vi "geterrormessages.vi"(8 "error in (no error)":errorcluster, 11 "hObject":i32=1) -> (0 "error out":errorcluster, 1 "pNumOfErrors":i32, 2 "pErrorMsgs":i32[](array[numeric]), 3 "hObject Out":i32=1)   [LabVIEW 2018]
doc: "This VI returns the errors from the neoVI error queue. Use \"GetErrorInfo\" to return the actual error info.\n\n12/21/2010 1.0.0 jyg\n- initial release"
uses:
  icsneo40.dll
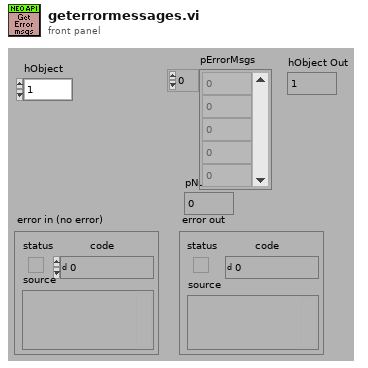
[diagram p1: front panel]
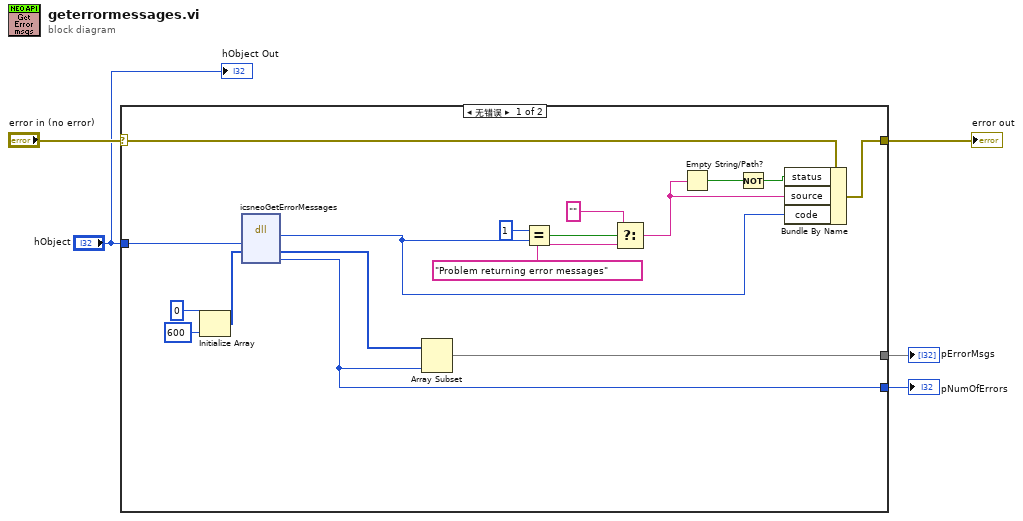
[diagram p0: block diagram]
diagram:
  n1 = case shown="无错误" "error in (no error)" {
    selector: "error in (no error)" -> [w19 w23]
    tunnel: [w20 w23] -> w5
    tunnel: [w16 _] -> w3
    tunnel: "hObject" -> [w15 _]
    tunnel: [w10 _] -> w2
    frame No Error {
      n2 = Initialize Array(0, 600 ("dimension size")) -> (w12:i32[])
      n3 = dll-call lib="icsneo40.dll" fn="icsneoGetErrorMessages"("hObject"=w15, "pErrorMsgs"=w12) -> ("return type"=w6:i32, "pErrorMsgs"=w11:i32[], "pNumOfErrors"=w16:i32)  [unwired: 4 in, 3 out]
      n4 = Array Subset(array=w11, length=w16) -> (w10:i32[])  [unwired: 1 in]
      n5 = Equal?(x=1, y=w6) -> (x = y?=w18:bool)
      n6 = Select(t="" ("f"), s=w18, f="Problem returning error messages") -> (s? t:f=w17:string)
      n7 = Empty String/Path?(string/path=w17) -> (empty?=w22:bool)
      n8 = Not(x=w22) -> (.not. x?=w21:bool)
      n9 = Bundle By Name(cluster=w19, "status"=w21, "source"=w17, "code"=w6) -> (w20:errorcluster)
    }
    frame Error {
    }
  }
  "error out" <- w5
  "pNumOfErrors" <- w3
  "pErrorMsgs" <- w2
  "hObject Out" <- "hObject"
